vi "Write outgoing label data.vi"(4 "ScheduledSDI":bool, 6 "Iteration":i32, 8 "error in (no error)":errorcluster, 9 "Last iteration values":dbl[](array[numeric]), 10 "This iteration values":dbl[](array[numeric]), 11 "Label Settings":T1 {"Words"."Param Setting"."Num Bits" min=1 max=32; "Words"."Param Setting"."Start Bit" min=8 max=31; "Words"."Block Data Refs"."Data Reference" format="%.0x"; "Label" format="%.0o"}) -> (0 "error out":errorcluster, 1 "Last iteration values Out":dbl[](array[numeric]), 3 "Label Settings":T1 {"Words"."Param Setting"."Num Bits" min=1 max=32; "Words"."Param Setting"."Start Bit" min=8 max=31; "Words"."Block Data Refs"."Data Reference" format="%.0x"; "Label" format="%.0o"})   [LabVIEW 2016, in "Ballard Arinc-429 Engine.lvlib"]
uses:
  Ballard Arinc-429 Engine.lvlib
  RT Controls/RT Label Settings.ctl
  Shared/Controls and Global/Label.ctl
  Shared/Controls and Global/transferPeriod.ctl
  RT Controls/Driver Data.ctl
  RT Controls/RT Word Settings.ctl
  <vilib>/NI Veristand/Custom Device API/Block Data Reference.ctl
  <vilib>/NI Veristand/Custom Device API/Data Reference.ctl
  RT Controls/RT Param Setting.ctl
  Shared/Controls and Global/Start Bit.ctl
  Shared/Controls and Global/Number of Bits.ctl
  Shared/Controls and Global/TransferType.ctl
  <instrlib>/AIT 429/AIT 429.lvlib
  Shared/Ballard Arinc-429 Shared.lvlib
  <vilib>/NI Veristand/Custom Device API/Custom Device API.lvlib
panel:
  in  "Array length":i32
  in  "Array index":i32
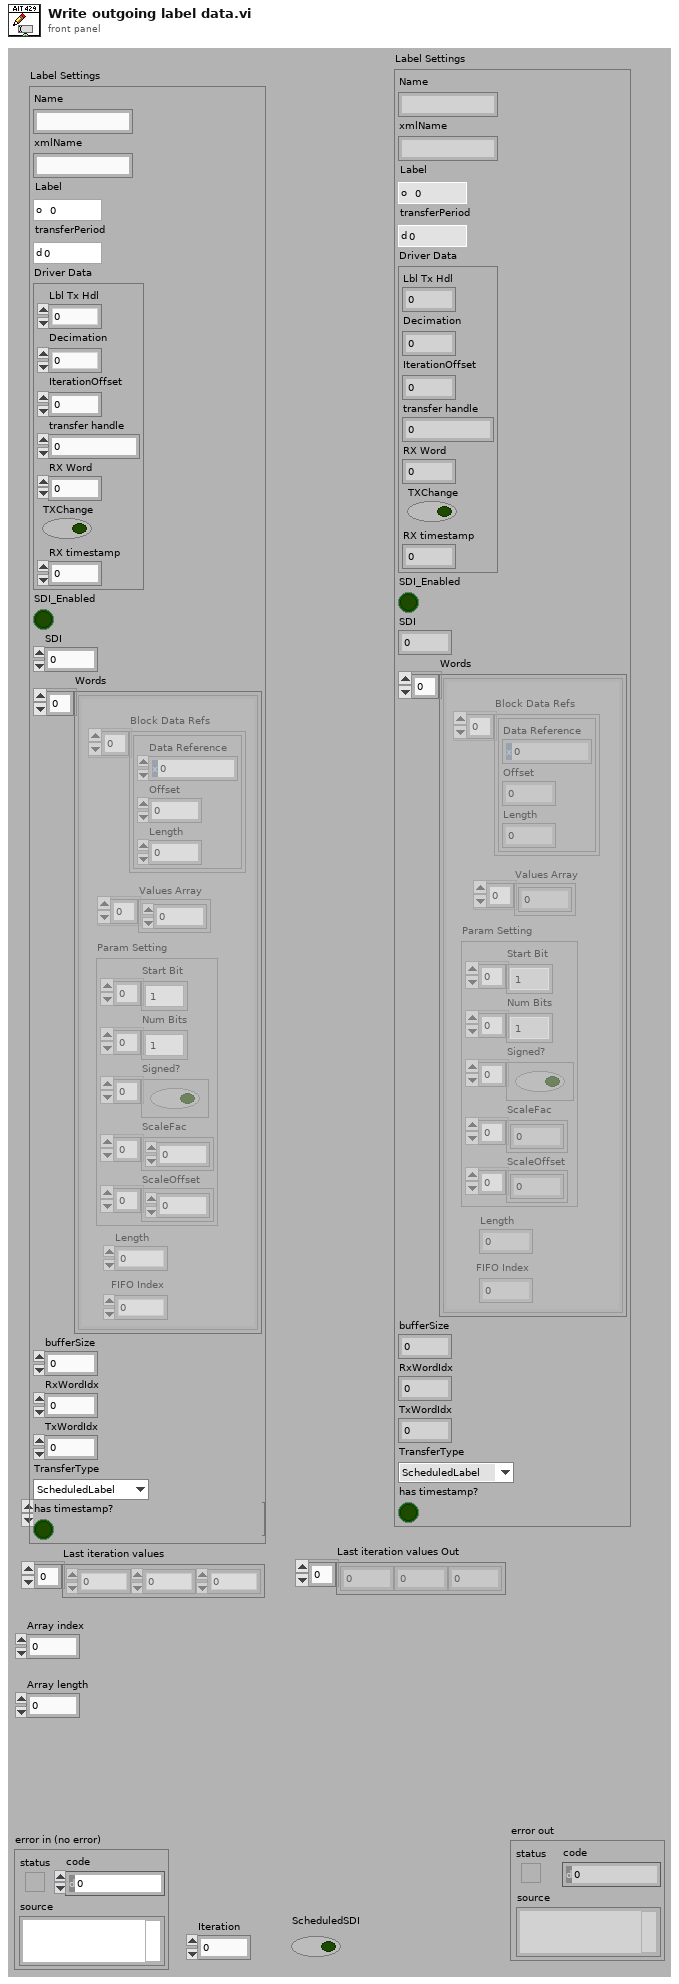
[diagram p1: front panel]
types:
  T1 = typedef "Ballard Arinc-429 Engine.lvlib/RT Label Settings.ctl" = cluster{"Name":string, "xmlName":string, "Label":T2, "transferPeriod":T3, "Driver Data":T4, "SDI_Enabled":bool, "SDI":u8, "Words":T5[], "bufferSize":u32, "RxWordIdx":i32, "TxWordIdx":i32, "TransferType":T11, "has timestamp?":bool}
  T2 = typedef "Ballard Arinc-429 Shared.lvlib/Label.ctl" = u8
  T3 = typedef "Ballard Arinc-429 Shared.lvlib/transferPeriod.ctl" = u32
  T4 = typedef "Ballard Arinc-429 Engine.lvlib/Driver Data.ctl" = cluster{"Lbl Tx Hdl":u32, "Decimation":i32, "IterationOffset":i32, "transfer handle":u32, "RX Word":u32, "TXChange":bool, "RX timestamp":dbl}
  T5 = typedef "Ballard Arinc-429 Engine.lvlib/RT Word Settings.ctl" = cluster{"Block Data Refs":T6[], "Values Array":dbl[], "Length":i32, "FIFO Index":i32, "Param Setting":T8}
  T6 = typedef "Custom Device API.lvlib/Block Data Reference.ctl" = cluster{"Data Reference":T7, "Offset":u64, "Length":u64}
  T7 = typedef "Custom Device API.lvlib/Data Reference.ctl" = i32
  T8 = typedef "Ballard Arinc-429 Engine.lvlib/RT Param Setting.ctl" = cluster{"Start Bit":T9[], "Num Bits":T10[], "Signed?":bool[], "ScaleFac":dbl[], "ScaleOffset":dbl[]}
  T9 = typedef "Ballard Arinc-429 Shared.lvlib/Start Bit.ctl" = i32
  T10 = typedef "Ballard Arinc-429 Shared.lvlib/Number of Bits.ctl" = i32
  T11 = typedef "Ballard Arinc-429 Shared.lvlib/TransferType.ctl" = enum16{"ScheduledLabel", "Acyclic", "Block", "Strobe"}
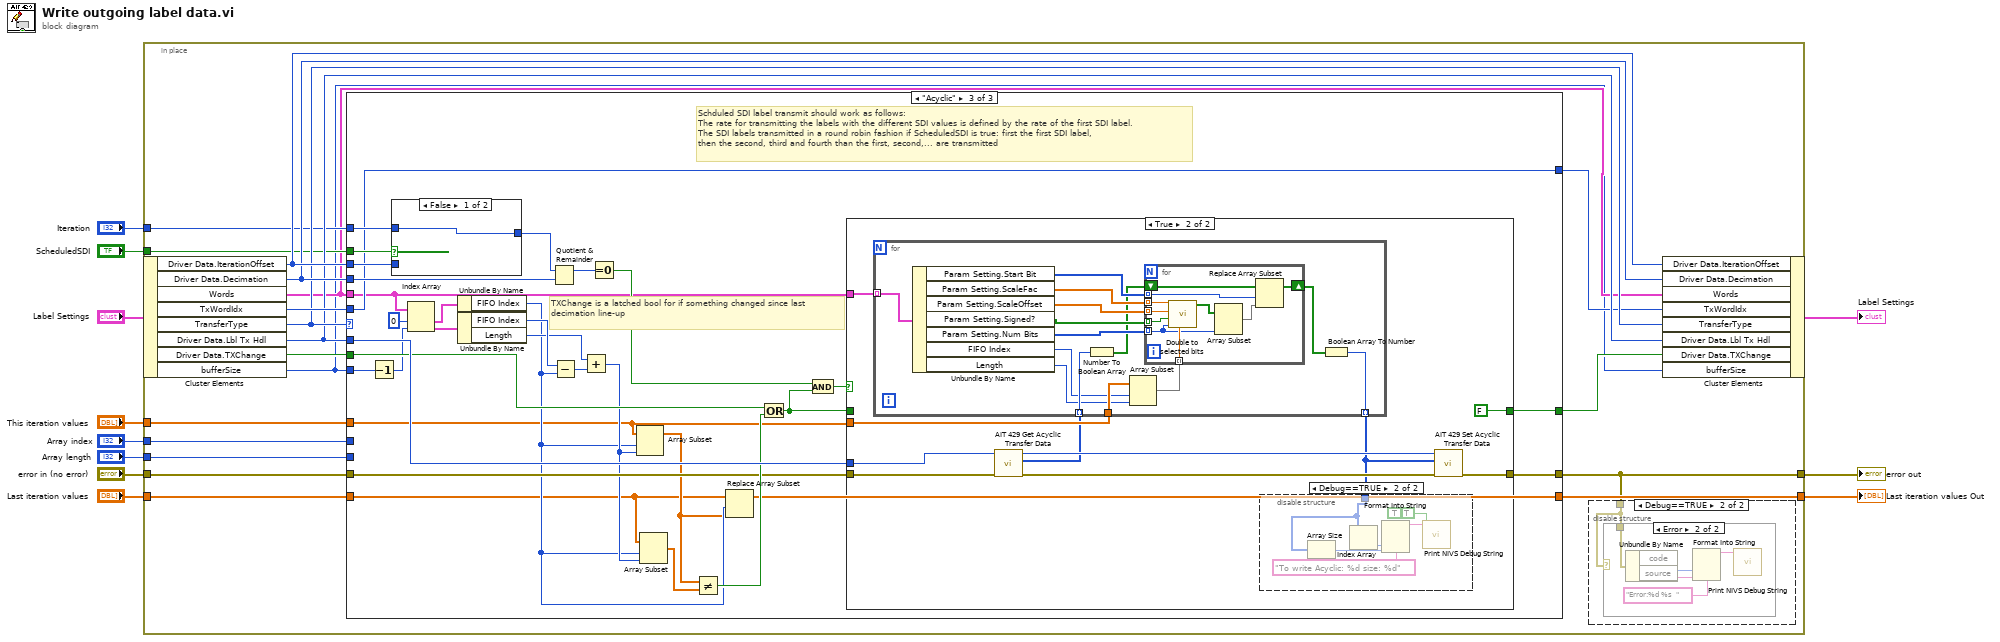
[diagram p0: block diagram]
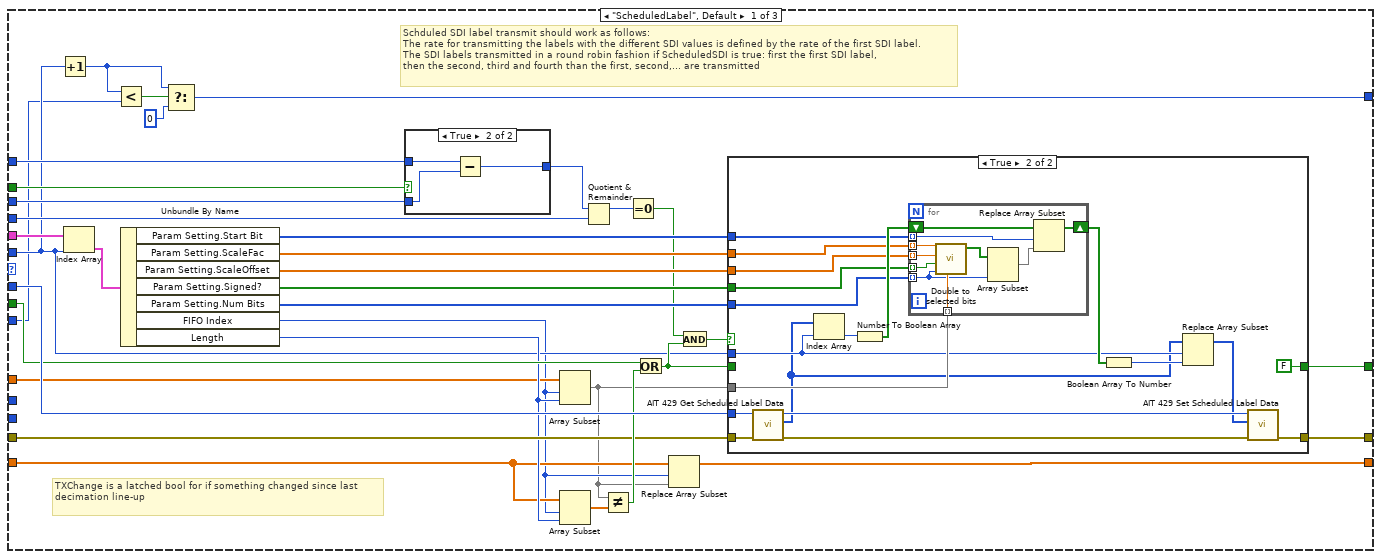
[diagram p4: hidden frame]
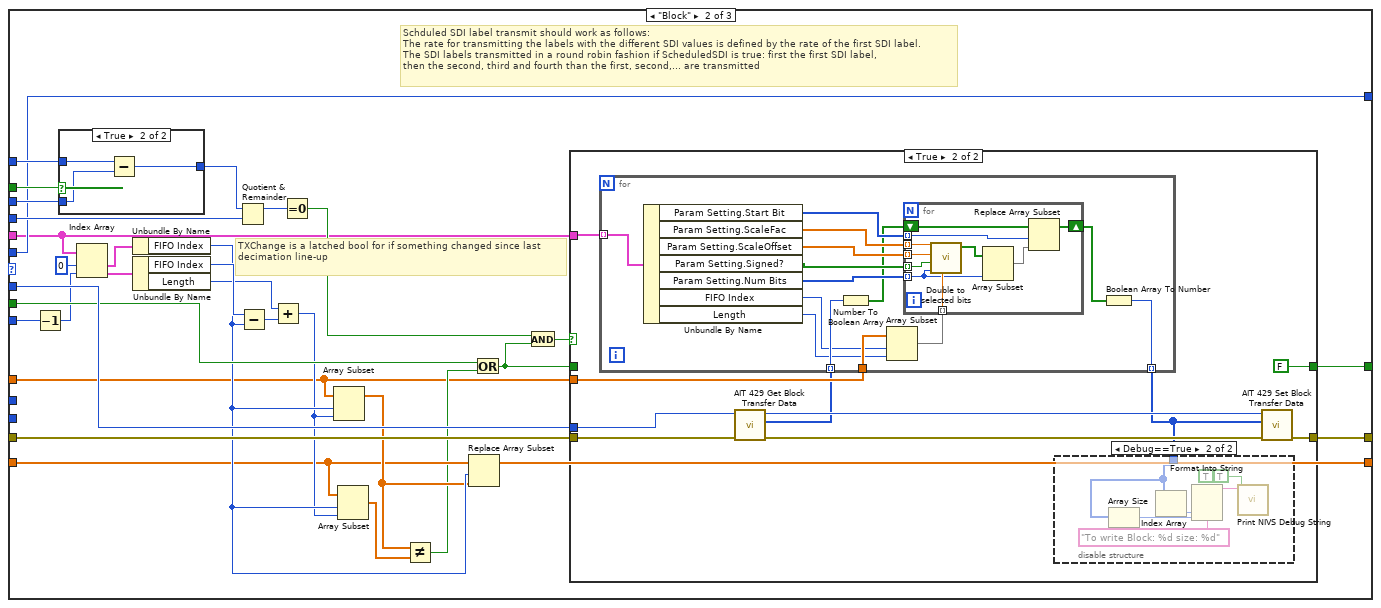
[diagram p7: hidden frame]
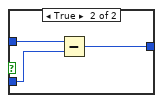
[diagram p13: hidden frame]
diagram:
  n1 = in-place {
    in-place-border: "This iteration values" -> [w27]
    in-place-border: "Array index" -> [w26]
    in-place-border: "Array length" -> [w25]
    in-place-border: "error in (no error)" -> [w24]
    in-place-border: "Last iteration values" -> [w23]
    in-place-border: [w12] -> w5
    in-place-border: "Iteration" -> [w18]
    in-place-border: "ScheduledSDI" -> [w17]
    in-place-border: [w14] -> w1
    n2 = in-place-cluster #1("Label Settings") -> ("Driver Data.IterationOffset"=w22:i32, "Driver Data.Decimation"=w21:i32, "Words"=w15:T5[], "TxWordIdx"=w30:i32, "TransferType"=w20:T11, "Driver Data.Lbl Tx Hdl"=w19:u32, "Driver Data.TXChange"=w29:bool, "bufferSize"=w13:u32)
    n3 = case shown="\"Acyclic\"" w20 {
      tunnel: w30 -> [w42 w124 w202]
      tunnel: w15 -> [w71 w123 w201]
      tunnel: w22 -> [w70 w138 w217]
      tunnel: w21 -> [w69 w137 w216]
      tunnel: w19 -> [w68 w136 w215]
      tunnel: w29 -> [w67 w135 w214]
      tunnel: [w66 w134 w213] -> w28
      tunnel: w27 -> [w44 w107 w186]
      tunnel: w26 -> [_ _ _]
      tunnel: w25 -> [_ _ _]
      tunnel: w24 -> [w53 w128 w206]
      tunnel: w23 -> [w40 w110 w187]
      tunnel: [w52 w127 w205] -> w12
      tunnel: w18 -> [w51 w126 w204]
      tunnel: w17 -> [w50 w125 w203]
      tunnel: [w47 w124 w202] -> w16
      tunnel: [w41 w114 w191] -> w14
      tunnel: w13 -> [w37 w121 w199]
      frame "ScheduledLabel", Default {
        # "TXChange is a latched bool for if something changed since last decimation line-up"
        # "Schduled SDI label transmit should work as follows:\nThe rate for transmitting the labels with the different SDI values is defined by the rate of the first SDI label.\nThe SDI labels transmitted in a round robin fashion if ScheduledSDI is true: first the first SDI label, \nthen the second, third and fourth than the first, second,... are transmitted"
        n4 = Increment(x=w42) -> (x+1=w45:i32)
        n5 = Index Array(array=w71, index=w42) -> (element=w65:T5)
        n6 = Less?(x=w45, y=w37) -> (x < y?=w49:bool)
        n7 = Unbundle By Name(w65) -> ("Param Setting.Start Bit"=w64:T9[], "Param Setting.ScaleFac"=w63:dbl[], "Param Setting.ScaleOffset"=w62:dbl[], "Param Setting.Signed?"=w61:bool[], "Param Setting.Num Bits"=w60:T10[], "FIFO Index"=w39:i32, "Length"=w46:i32)
        n8 = Select(t=w45, s=w49, f=0 ("TxWordIdx")) -> (s? t:f=w47:i32)
        n9 = case shown="True" w50 {
          tunnel: w51 -> [w103 w104]
          tunnel: [w103 w106] -> w58
          tunnel: w70 -> [_ w105]
          frame False {
          }
          frame True {
            n10 = Subtract(x=w104, y=w105) -> (x-y=w106:i32)
          }
        }
        n11 = Array Subset(array=w44, index=w39, length=w46) -> (w38:dbl[])
        n12 = Array Subset(array=w40, index=w39, length=w46) -> (w43:dbl[])
        n13 = Quotient & Remainder(x=w58, y=w69) -> (x-y*floor(x/y)=w59:i32)  [unwired: 1 out]
        n14 = Not Equal?(x=w38, y=w43) -> (x != y?=w57:bool)
        n15 = Equal To 0?(x=w59) -> (x = 0?=w56:bool)
        n16 = Or(x=w67, y=w57) -> (x .or. y?=w54:bool)
        n17 = Replace Array Subset(array=w40, new element=w38, index=w39) -> (w41:dbl[])
        n18 = And(x=w56, y=w54) -> (x .and. y?=w55:bool)
        n19 = case shown="True" w55 {
          tunnel: w64 -> [_ w89]
          tunnel: w60 -> [_ w90]
          tunnel: [w73 w80] -> w52
          tunnel: w53 -> [w73 w84]
          tunnel: w68 -> [_ w83]
          tunnel: w63 -> [_ w88]
          tunnel: w62 -> [_ w87]
          tunnel: w61 -> [_ w86]
          tunnel: w38 -> [_ w85]
          tunnel: w54 -> [w72 _]
          tunnel: [w72 FALSE] -> w66
          tunnel: w42 -> [_ w77]
          frame False {
          }
          frame True {
            (unwired) FALSE
            n20 = call <instrlib>:"AIT 429 Get Scheduled Label Data.vi"("error in (no error)"=w84, "scheduled label handle"=w83) -> ("error out"=w81:errorcluster, "word array"=w76:u32[], "scheduled label handle"=w79:u64)  [unwired: 7 in]
            n21 = Index Array(array=w76, index=w77) -> (element=w82:u32)
            n22 = Number To Boolean Array(number=w82) -> (Boolean array=w92:bool[])
            n23 = for {
              tunnel: w89 -> [w101] mode=indexing
              tunnel: w90 -> [w96] mode=indexing
              tunnel: w85 -> [w97] mode=indexing
              shift-right: [w99] -> w91
              shift-left: w92 -> [w102]
              tunnel: w88 -> [w95] mode=indexing
              tunnel: w87 -> [w94] mode=indexing
              tunnel: w86 -> [w93] mode=indexing
              n24 = call "Double to selected bits.vi"("Double"=w97, "Number of Bits"=w96, "Signed?"=w93, "ScaleOffset"=w94, "ScaleFac"=w95) -> ("Bits"=w98:bool[])  [unwired: 6 in]
              n25 = Array Subset(array=w98, length=w96) -> (w100:bool[])  [unwired: 1 in]
              n26 = Replace Array Subset(array=w102, new element=w100, index=w101) -> (w99:bool[])
            }
            n27 = Boolean Array To Number(Boolean array=w91) -> (number=w78:u32)
            n28 = Replace Array Subset(array=w76, new element=w78, index=w77) -> (w75:u32[])
            n29 = call <instrlib>:"AIT 429 Set Scheduled Label Data.vi"("error in (no error)"=w81, "word array"=w75, "scheduled label handle"=w79) -> ("error out"=w80:errorcluster)  [unwired: 6 in, 2 out]
          }
        }
      }
      frame "Block" {
        # "TXChange is a latched bool for if something changed since last decimation line-up"
        # "Schduled SDI label transmit should work as follows:\nThe rate for transmitting the labels with the different SDI values is defined by the rate of the first SDI label.\nThe SDI labels transmitted in a round robin fashion if ScheduledSDI is true: first the first SDI label, \nthen the second, third and fourth than the first, second,... are transmitted"
        n30 = Decrement(x=w121) -> (x-1=w120:u32)
        n31 = case shown="True" w125 {
          tunnel: w126 -> [w182 w183]
          tunnel: [w182 w185] -> w132
          tunnel: w138 -> [_ w184]
          frame False {
          }
          frame True {
            n32 = Subtract(x=w183, y=w184) -> (x-y=w185:i32)
          }
        }
        n33 = Index Array(array=w123, index #1=0 ("index"), index #2=w120) -> (element #1=w119:T5, element #2=w118:T5)
        n34 = Unbundle By Name(w119) -> ("FIFO Index"=w113:i32)
        n35 = Unbundle By Name(w118) -> ("FIFO Index"=w117:i32, "Length"=w115:i32)
        n36 = Quotient & Remainder(x=w132, y=w137) -> (x-y*floor(x/y)=w133:i32)  [unwired: 1 out]
        n37 = Subtract(x=w117, y=w113) -> (x-y=w116:i32)
        n38 = Add(x=w115, y=w116) -> (x+y=w112:i32)
        n39 = Equal To 0?(x=w133) -> (x = 0?=w131:bool)
        n40 = Array Subset(array=w107, index=w113, length=w112) -> (w111:dbl[])
        n41 = Array Subset(array=w110, index=w113, length=w112) -> (w109:dbl[])
        n42 = Not Equal?(x=w111, y=w109) -> (x != y?=w108:bool)
        n43 = Replace Array Subset(array=w110, new element=w111, index=w113) -> (w114:dbl[])
        n44 = Or(x=w135, y=w108) -> (x .or. y?=w129:bool)
        n45 = And(x=w131, y=w129) -> (x .and. y?=w130:bool)
        n46 = case shown="True" w130 {
          tunnel: [w140 w145] -> w127
          tunnel: w128 -> [w140 w147]
          tunnel: w136 -> [_ w144]
          tunnel: w107 -> [_ w148]
          tunnel: w129 -> [w139 _]
          tunnel: [w139 FALSE] -> w134
          tunnel: w123 -> [_ w149]
          frame False {
          }
          frame True {
            n47 = call <instrlib>:"AIT 429 Get Block Transfer Data.vi"("error in"=w147, "block transfer handle in"=w144) -> ("error out"=w146:errorcluster, "word array out"=w142:u32[], "block transfer handle out"=w143:u64)  [unwired: 7 in]
            n48 = for {
              tunnel: w148 -> [w161]
              tunnel: [w170] -> w141 mode=indexing
              tunnel: w149 -> [w164] mode=indexing
              tunnel: w142 -> [w162] mode=indexing
              n49 = Unbundle By Name(w164) -> ("Param Setting.Start Bit"=w169:T9[], "Param Setting.ScaleFac"=w168:dbl[], "Param Setting.ScaleOffset"=w167:dbl[], "Param Setting.Signed?"=w166:bool[], "Param Setting.Num Bits"=w165:T10[], "FIFO Index"=w160:i32, "Length"=w159:i32)
              n50 = Number To Boolean Array(number=w162) -> (Boolean array=w163:bool[])
              n51 = Array Subset(array=w161, index=w160, length=w159) -> (w158:dbl[])
              n52 = for {
                tunnel: w169 -> [w180] mode=indexing
                tunnel: w165 -> [w175] mode=indexing
                tunnel: w158 -> [w176] mode=indexing
                shift-right: [w178] -> w171
                shift-left: w163 -> [w181]
                tunnel: w168 -> [w174] mode=indexing
                tunnel: w167 -> [w173] mode=indexing
                tunnel: w166 -> [w172] mode=indexing
                n53 = call "Double to selected bits.vi"("Double"=w176, "Number of Bits"=w175, "Signed?"=w172, "ScaleOffset"=w173, "ScaleFac"=w174) -> ("Bits"=w177:bool[])  [unwired: 6 in]
                n54 = Array Subset(array=w177, length=w175) -> (w179:bool[])  [unwired: 1 in]
                n55 = Replace Array Subset(array=w181, new element=w179, index=w180) -> (w178:bool[])
              }
              n56 = Boolean Array To Number(Boolean array=w171) -> (number=w170:u32)
            }
            n57 = disable-structure shown="Debug==True" {
              disable-tunnel: w141 -> [_ w151]
              frame condition #0 (active) {
              }
              frame condition #1 {
                n58 = Array Size(array=w151) -> (size(s)=w152:i32)
                n59 = Index Array(array=w151) -> (element=w154:u32)  [unwired: 1 in]
                n60 = Format Into String(format string="To write Block: %d size: %d", w154, w152) -> (resulting string=w157:string)  [unwired: 2 in, 1 out]
                n61 = call "Print NIVS Debug String.vi"("Add to NIVS Log FIle? (T)"=TRUE, "Append EOL? (T)"=TRUE, "Debug String"=w157) -> ()  [unwired: 7 in, 1 out]
              }
            }
            n62 = call <instrlib>:"AIT 429 Set Block Transfer Data.vi"("error in (no error)"=w146, "word array"=w141, "block transfer handle in"=w143) -> ("error out"=w145:errorcluster)  [unwired: 6 in, 2 out]
          }
        }
      }
      frame "Acyclic" {
        # "TXChange is a latched bool for if something changed since last decimation line-up"
        # "Schduled SDI label transmit should work as follows:\nThe rate for transmitting the labels with the different SDI values is defined by the rate of the first SDI label.\nThe SDI labels transmitted in a round robin fashion if ScheduledSDI is true: first the first SDI label, \nthen the second, third and fourth than the first, second,... are transmitted"
        n63 = Decrement(x=w199) -> (x-1=w198:u32)
        n64 = case shown="False" w203 {
          tunnel: w204 -> [w261 w262]
          tunnel: [w261 w264] -> w211
          tunnel: w217 -> [_ w263]
          frame False {
          }
          frame True {
            n65 = Subtract(x=w262, y=w263) -> (x-y=w264:i32)
          }
        }
        n66 = Index Array(array=w201, index #1=0 ("index"), index #2=w198) -> (element #1=w197:T5, element #2=w196:T5)
        n67 = Unbundle By Name(w197) -> ("FIFO Index"=w190:i32)
        n68 = Unbundle By Name(w196) -> ("FIFO Index"=w195:i32, "Length"=w193:i32)
        n69 = Quotient & Remainder(x=w211, y=w216) -> (x-y*floor(x/y)=w212:i32)  [unwired: 1 out]
        n70 = Subtract(x=w195, y=w190) -> (x-y=w194:i32)
        n71 = Add(x=w193, y=w194) -> (x+y=w192:i32)
        n72 = Equal To 0?(x=w212) -> (x = 0?=w209:bool)
        n73 = Array Subset(array=w186, index=w190, length=w192) -> (w189:dbl[])
        n74 = Array Subset(array=w187, index=w190, length=w192) -> (w188:dbl[])
        n75 = Not Equal?(x=w189, y=w188) -> (x != y?=w210:bool)
        n76 = Replace Array Subset(array=w187, new element=w189, index=w190) -> (w191:dbl[])
        n77 = Or(x=w214, y=w210) -> (x .or. y?=w207:bool)
        n78 = And(x=w209, y=w207) -> (x .and. y?=w208:bool)
        n79 = case shown="True" w208 {
          tunnel: [w219 w221] -> w205
          tunnel: w206 -> [w219 w223]
          tunnel: w215 -> [_ w226]
          tunnel: w186 -> [_ w227]
          tunnel: w207 -> [w218 _]
          tunnel: [w218 FALSE] -> w213
          tunnel: w201 -> [_ w228]
          frame False {
          }
          frame True {
            n80 = call <instrlib>:"AIT 429 Get Acyclic Transfer Data.vi"("error in (no error)"=w223, "transfer handle"=w226) -> ("error out"=w222:errorcluster, "word array"=w224:u32[], "transfer handle"=w225:u64)  [unwired: 7 in]
            n81 = for {
              tunnel: w227 -> [w240]
              tunnel: [w249] -> w220 mode=indexing
              tunnel: w228 -> [w243] mode=indexing
              tunnel: w224 -> [w241] mode=indexing
              n82 = Unbundle By Name(w243) -> ("Param Setting.Start Bit"=w248:T9[], "Param Setting.ScaleFac"=w247:dbl[], "Param Setting.ScaleOffset"=w246:dbl[], "Param Setting.Signed?"=w245:bool[], "Param Setting.Num Bits"=w244:T10[], "FIFO Index"=w239:i32, "Length"=w238:i32)
              n83 = Number To Boolean Array(number=w241) -> (Boolean array=w242:bool[])
              n84 = Array Subset(array=w240, index=w239, length=w238) -> (w237:dbl[])
              n85 = for {
                tunnel: w248 -> [w259] mode=indexing
                tunnel: w244 -> [w254] mode=indexing
                tunnel: w237 -> [w255] mode=indexing
                shift-right: [w257] -> w250
                shift-left: w242 -> [w260]
                tunnel: w247 -> [w253] mode=indexing
                tunnel: w246 -> [w252] mode=indexing
                tunnel: w245 -> [w251] mode=indexing
                n86 = call "Double to selected bits.vi"("Double"=w255, "Number of Bits"=w254, "Signed?"=w251, "ScaleOffset"=w252, "ScaleFac"=w253) -> ("Bits"=w256:bool[])  [unwired: 6 in]
                n87 = Array Subset(array=w256, length=w254) -> (w258:bool[])  [unwired: 1 in]
                n88 = Replace Array Subset(array=w260, new element=w258, index=w259) -> (w257:bool[])
              }
              n89 = Boolean Array To Number(Boolean array=w250) -> (number=w249:u32)
            }
            n90 = disable-structure shown="Debug==TRUE" {
              disable-tunnel: w220 -> [_ w230]
              frame condition #0 (active) {
              }
              frame condition #1 {
                n91 = Array Size(array=w230) -> (size(s)=w231:i32)
                n92 = Index Array(array=w230) -> (element=w233:u32)  [unwired: 1 in]
                n93 = Format Into String(format string="To write Acyclic: %d size: %d", w233, w231) -> (resulting string=w236:string)  [unwired: 2 in, 1 out]
                n94 = call "Print NIVS Debug String.vi"("Add to NIVS Log FIle? (T)"=TRUE, "Append EOL? (T)"=TRUE, "Debug String"=w236) -> ()  [unwired: 7 in, 1 out]
              }
            }
            n95 = call <instrlib>:"AIT 429 Set Acyclic Transfer Data.vi"("error in (no error)"=w222, "word array"=w220, "transfer handle"=w225) -> ("error out"=w221:errorcluster)  [unwired: 7 in, 1 out]
          }
        }
      }
    }
    n96 = disable-structure shown="Debug==TRUE" {
      disable-tunnel: w12 -> [_ w31]
      frame condition #0 (active) {
      }
      frame condition #1 {
        n97 = case shown="Error" w31 {
          tunnel: w31 -> [_ w34]
          frame No Error {
          }
          frame Error {
            n98 = Unbundle By Name(w34) -> ("code"=w33:i32, "source"=w32:string)
            n99 = Format Into String(format string="Error:%d %s  ", w33, w32) -> (resulting string=w35:string)  [unwired: 2 in, 1 out]
            n100 = call "Print NIVS Debug String.vi"("Debug String"=w35) -> ()  [unwired: 9 in, 1 out]
          }
        }
      }
    }
    n101 = in-place-cluster #1("Driver Data.IterationOffset"=w22, "Driver Data.Decimation"=w21, "Words"=w15, "TxWordIdx"=w16, "TransferType"=w20, "Driver Data.Lbl Tx Hdl"=w19, "Driver Data.TXChange"=w28, "bufferSize"=w13) -> (→"Label Settings":T1)
  }
  "error out" <- w5
  "Last iteration values Out" <- w1
